vi "Perform Action.vi"(7 "Instrument":refnum<class "Instrument.lvclass">, 8 "error in":errorcluster, 10 "Input":variant, 11 "object in":refnum<class "Perform Action Remote on Const Channel with 3DBL Strategy.lvclass">) -> (0 "error out":errorcluster, 2 "Output":variant, 3 "object out":refnum<class "Perform Action Remote on Const Channel with 3DBL Strategy.lvclass">)   [LabVIEW 2023, in "HAL.lvlib" / "Perform Action Remote on Const Channel with 3DBL Strategy.lvclass"]
uses:
  Perform Action Remote on Const Channel with 3DBL Strategy.lvclass
  Perform Action Remote on Const Channel with 3DBL Strategy.lvclass/Perform Action Remote on Const Channel with 3DBL Strategy.ctl
  PA on Const Channel Strategy/Perform Action on Const Channel Strategy.lvclass
  Instrument/Instrument.lvclass
  D:/git/HAL/HAL/Virtual Instruments/PA on Const Channel Strategy/Perform Action on Const Channel Strategy.lvclass
  D:/git/HAL/HAL/Virtual Instruments/Perform Action Strategy/Perform Action Strategy.lvclass
  D:/git/HAL/HAL/Virtual Instruments/PA Remote on Const Channel with 3DBL Strategy/Perform Action Remote on Const Channel with 3DBL Strategy.lvclass
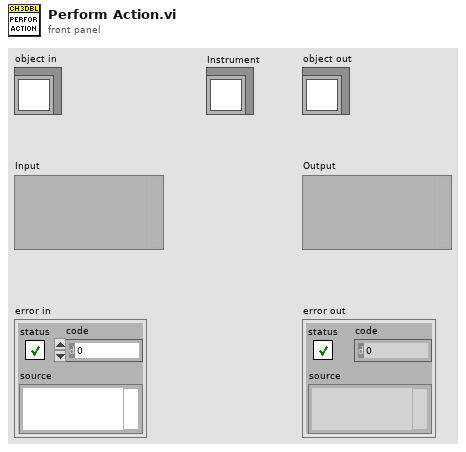
[diagram p1: front panel]
types:
  T1 = cluster{"Channel":string, cluster{dbl, dbl, dbl}}
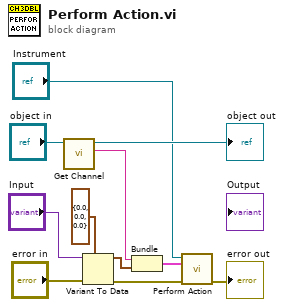
[diagram p0: block diagram]
diagram:
  n1 = call "Get Channel.vi"("Perform Action on Const Channel Strategy in"="object in") -> ("Channel"=w2:string, "Perform Action on Const Channel Strategy out"=→"object out":refnum<class "Perform Action Remote on Const Channel with 3DBL Strategy.lvclass">)  [unwired: 9 in]
  n2 = Variant To Data(error in="error in", type=cluster{dbl, dbl, dbl} {0.0, 0.0, 0.0}, Variant="Input") -> (data=w10:cluster{dbl, dbl, dbl}, error out=w11:errorcluster)
  n3 = Bundle("Channel"=w2, w10) -> (w9:T1)  [unwired: 1 in]
  n4 = call "Perform Action.vi"("Error In"=w11, "Input"=w9, "reference in"="Instrument") -> ("Error Out"=→"error out":errorcluster)  [unwired: 6 in, 2 out]
